vi "Drive for Time.vi"(6 "Synchronization":enum16{"Start", "Wait"}(ring), 7 "Description":string, 8 "Command Info In":T1, 9 "Seconds":dbl, 10 "Right Speed":dbl, 11 "Left Speed":dbl) -> (0 "Command Info Out":T1)   [LabVIEW 2020]
doc: "This VI sets the motors to run for a given number of seconds. It optionally synchronizes with the completion of the command."
uses:
  <vilib>/Rock Robotics/WPI/Framework/Command Status Info.ctl
  <vilib>/Rock Robotics/WPI/Framework/Completion Status.ctl
  <vilib>/Rock Robotics/WPI/Framework/Completion Notifier.ctl
  Implementation/Drive Setpoints.ctl
  Implementation/Drive Operations.ctl
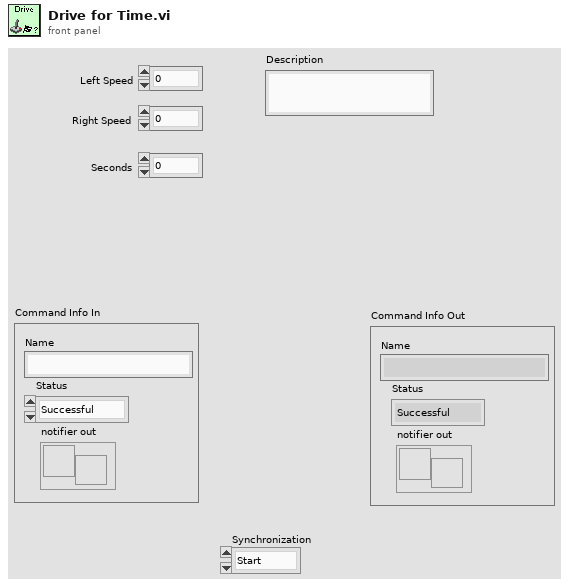
[diagram p1: front panel]
types:
  T1 = typedef "Command Status Info.ctl" = cluster{"Name":string, "Status":T2, "notifier out":T3}
  T2 = typedef "Completion Status.ctl" = enum16{"Successful", "Aborted", "Incomplete"}
  T3 = typedef "Completion Notifier.ctl" = refnum<notifier>
  T4 = typedef "Drive Setpoints.ctl" = cluster{"Operation":T5, "Left Joystick X-Axis":dbl, "Left Joystick Y-Axis":dbl, "Duration":dbl, "Right Joystick Y-Axis":dbl, "Right Joystick X-Axis":dbl}
  T5 = typedef "Drive Operations.ctl" = enum16{"Reserve", "Read Current", "Rocket Drive Immediate", "Tank Drive Immediate", "Drive for Time", "Drive for Distance"}
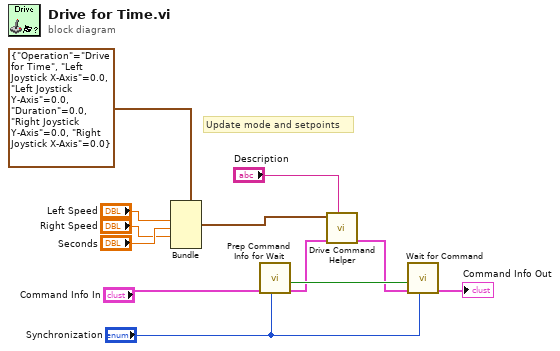
[diagram p0: block diagram]
diagram:
  # "Update mode and setpoints"
  n1 = Bundle(cluster=T4 {"Operation"=enum."Drive for Time", "Left Joystick X-Axis"=0.0, "Left Joystick Y-Axis"=0.0, "Duration"=0.0, "Right Joystick Y-Axis"=0.0, "Right Joystick X-Axis"=0.0} ("SubSystem Data"), "Left Joystick Y-Axis"="Left Speed", "Duration"="Seconds", "Right Joystick Y-Axis"="Right Speed") -> (w5:T4)  [unwired: 3 in]
  n2 = call <vilib>:"Prep Command Info for Wait.vi"("Synchronication"="Synchronization", "Command Info"="Command Info In") -> ("Command Info"=w9:T1, "Allocated"=w10:bool)  [unwired: 8 in]
  n3 = call "Drive Command Helper.vi"("Description"="Description", "Command Info In"=w9, "SubSystem Data"=w5) -> ("Command Info Out"=w6:T1)  [unwired: 6 in, 2 out]
  n4 = call <vilib>:"Wait for Command.vi"("Synchronication"="Synchronization", "Command Info in"=w6, "Allocated"=w10) -> ("Command Info out"=→"Command Info Out":T1)  [unwired: 8 in]
